vi "PathPlanner_TrajectoryState_New.vi"(0 "PathPlannerConstraints":T1={"MaxVelocityMps;"=0.0, "MaxAccelerationMpsSq;"=0.0, "MaxAngularVelRadPsEc;"=0.0, "MaxAngularAccRadPSecSq"=0.0, "Exists"=FALSE, "Unlimited"=FALSE, "NominalVoltageVolts"=12.0}, 1 "WaypointRelPos":dbl, 3 "DeltaPos":dbl, 4 "CurvatureRadPerMeter":dbl, 5 "TimeSeconds":dbl, 6 "TargetHolonomicRotation":T2={"VALUE"=0.0, "COS"=1.0, "SIN"=0.0} {"SIN" format="%13.4f"; "COS" format="%13.4f"; "VALUE" format="%13.4f"}, 7 "VelocityMPS":dbl, 8 "Heading":T2={"VALUE"=0.0, "COS"=1.0, "SIN"=0.0} {"SIN" format="%13.4f"; "COS" format="%13.4f"; "VALUE" format="%13.4f"}, 9 "PositionMeters":T3 {"Y" format="%14.3f"; "X" format="%14.3f"}, 10 "HeadingAngularVelRadPerSec":dbl, 11 "AccerationMpsSq":dbl) -> (2 "PathPlannerState":T4={"TimeSeconds"=0.0, "VelocityMPS"=0.0, "AccerationMpsSq"=0.0, "HeadingAngularVelRadPerSec"=0.0, "PositionMeters"={"X"=0.0, "Y"=1.0}, "Heading"={"VALUE"=0.0, "COS"=1.0, "SIN"=0.0}, "TargetHolonomicRotation"={"VALUE"=0.0, "COS"=1.0, "SIN"=0.0}, "CurvatureRadPerMeter"=0.0, "PathPlannerConstraints"={"MaxVelocityMps;"=0.0, "MaxAccelerationMpsSq;"=0.0, "MaxAngularVelRadPsEc;"=0.0, "MaxAngularAccRadPSecSq"=0.0, "Exists"=FALSE, "Unlimited"=FALSE, "NominalVoltageVolts"=12.0}, "DeltaPos"=0.0, "WaypointRelPos"=0.0} {"TargetHolonomicRotation"."SIN" format="%13.4f"; "TargetHolonomicRotation"."COS" format="%13.4f"; "TargetHolonomicRotation"."VALUE" format="%13.4f"; "Heading"."SIN" format="%13.4f"; "Heading"."COS" format="%13.4f"; "Heading"."VALUE" format="%13.4f"; "PositionMeters"."Y" format="%14.3f"; "PositionMeters"."X" format="%14.3f"})   [LabVIEW 2019, in "PathPlanner24.lvlib"]
doc: "Create a trajectory state\n\nInputs:\n -- timeSeconds - double - The time at this state in seconds ( default = 0; )\n -- velocityMps - double - The velocity at this state in m/s ( default = 0 )\n -- accelerationMpsSq - double - The acceleration at this state in m/s^2 ( default = 0 )\n -- headingAngularVelocityRps - double - The time at this state in seconds ( default = 0 )\n -- positionMeters - translation2d - The position at this state in meters ( default = 0,0 )\n -- heading - rotation2d - The heading (direction of travel) at this state ( default = 0 )\n -- targetHolonomicRotation - rotation2d - The target holonomic rotation at this state ( default = 0 )\n -- curvatureRadPerMeter - double - The curvature at this state in rad/m ( default = 0 )\n -- constraints -- cluster -- constraints to apply at this state (default - none )\n\n\nOutputs\n - PathPlannerTrajectoryState -- cluster -- Newly created state"
uses:
  PathPlanner24.lvlib
  TypeDef/PathPlannerTrajectoryState.ctl
  <vilib>/Rock Robotics/WPI/ThirdParty/JAS_Junk/TrajLib/TypeDef/TRANSLATION2D.ctl
  <vilib>/Rock Robotics/WPI/ThirdParty/JAS_Junk/TrajLib/TypeDef/ROTATION2D.ctl
  TypeDef/PathPlannerPathConstraints.ctl
  <vilib>/Rock Robotics/WPI/ThirdParty/JAS_Junk/TrajLib/Trajectory_Library.lvlib
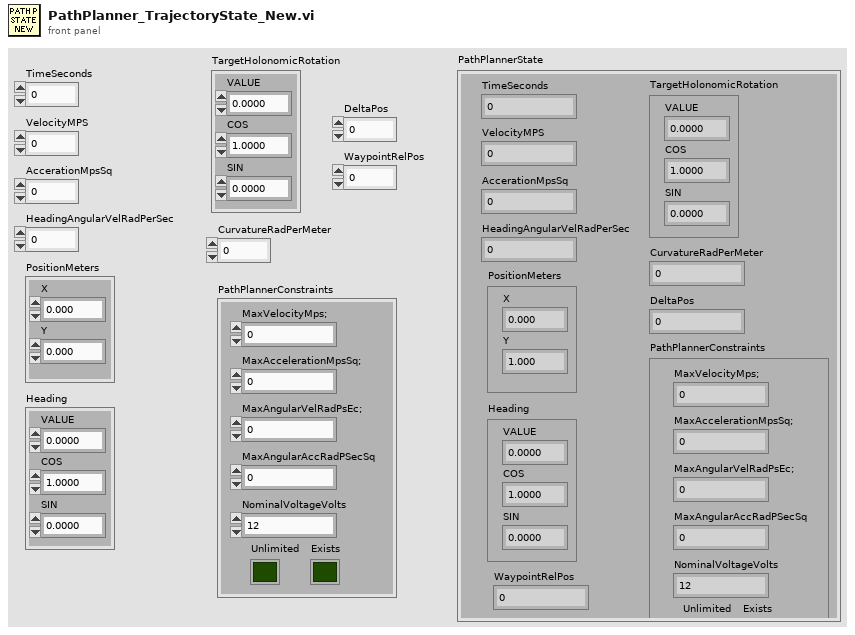
[diagram p1: front panel]
types:
  T1 = typedef "PathPlanner24.lvlib/PathPlannerPathConstraints.ctl" = cluster{"MaxVelocityMps;":dbl, "MaxAccelerationMpsSq;":dbl, "MaxAngularVelRadPsEc;":dbl, "MaxAngularAccRadPSecSq":dbl, "Exists":bool, "Unlimited":bool, "NominalVoltageVolts":dbl}
  T2 = typedef "Trajectory_Library.lvlib/ROTATION2D.ctl" = cluster{"VALUE":dbl, "COS":dbl, "SIN":dbl}
  T3 = typedef "Trajectory_Library.lvlib/TRANSLATION2D.ctl" = cluster{"X":dbl, "Y":dbl}
  T4 = typedef "PathPlanner24.lvlib/PathPlannerTrajectoryState.ctl" = cluster{"TimeSeconds":dbl, "VelocityMPS":dbl, "AccerationMpsSq":dbl, "HeadingAngularVelRadPerSec":dbl, "PositionMeters":T3, "Heading":T2, "TargetHolonomicRotation":T2, "CurvatureRadPerMeter":dbl, "PathPlannerConstraints":T1, "DeltaPos":dbl, "WaypointRelPos":dbl}
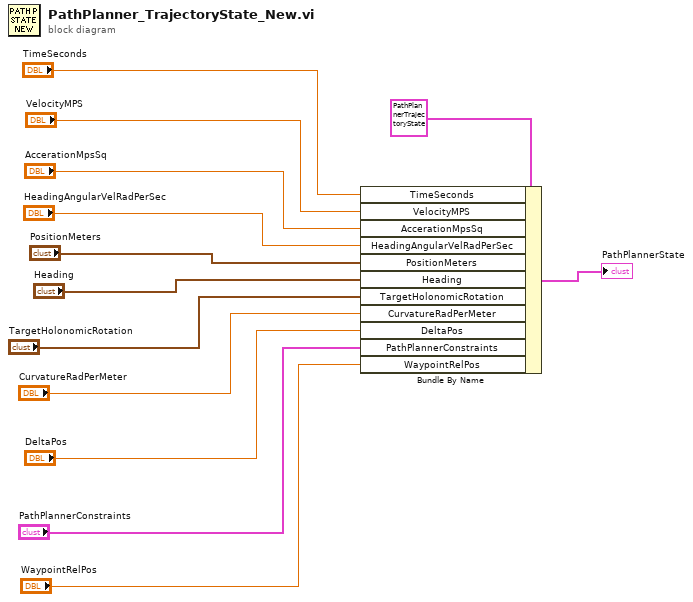
[diagram p0: block diagram]
diagram:
  n1 = Bundle By Name(cluster=T4 {"TimeSeconds"=0.0, "VelocityMPS"=0.0, "AccerationMpsSq"=0.0, "HeadingAngularVelRadPerSec"=0.0, "PositionMeters"={"X"=0.0, "Y"=1.0}, "Heading"={"VALUE"=0.0, "COS"=1.0, "SIN"=0.0}, "TargetHolonomicRotation"={"VALUE"=0.0, "COS"=1.0, "SIN"=0.0}, "CurvatureRadPerMeter"=0.0, "PathPlannerConstraints"={"MaxVelocityMps;"=0.0, "MaxAccelerationMpsSq;"=0.0, "MaxAngularVelRadPsEc;"=0.0, "MaxAngularAccRadPSecSq"=0.0, "Exists"=FALSE, "Unlimited"=FALSE, "NominalVoltageVolts"=12.0}, "DeltaPos"=0.0, "WaypointRelPos"=0.0} ("PathPlannerState"), "TimeSeconds"="TimeSeconds", "VelocityMPS"="VelocityMPS", "AccerationMpsSq"="AccerationMpsSq", "HeadingAngularVelRadPerSec"="HeadingAngularVelRadPerSec", "PositionMeters"="PositionMeters", "Heading"="Heading", "TargetHolonomicRotation"="TargetHolonomicRotation", "CurvatureRadPerMeter"="CurvatureRadPerMeter", "DeltaPos"="DeltaPos", "PathPlannerConstraints"="PathPlannerConstraints", "WaypointRelPos"="WaypointRelPos") -> (→"PathPlannerState":T4)
